vi "insertionSort.vi"() -> ()   [LabVIEW 2014]
panel:
  out "Insertion Sort":dbl[](graph)
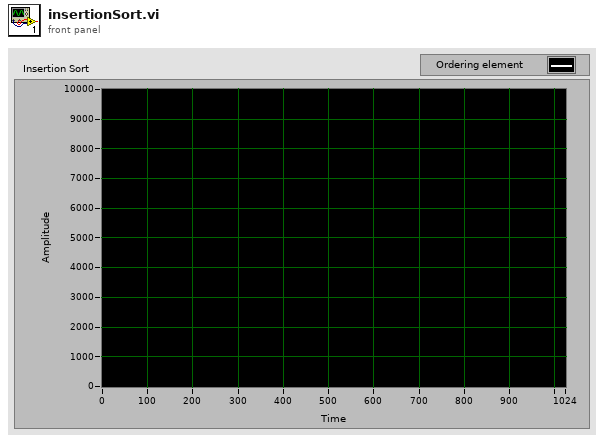
[diagram p1: front panel]
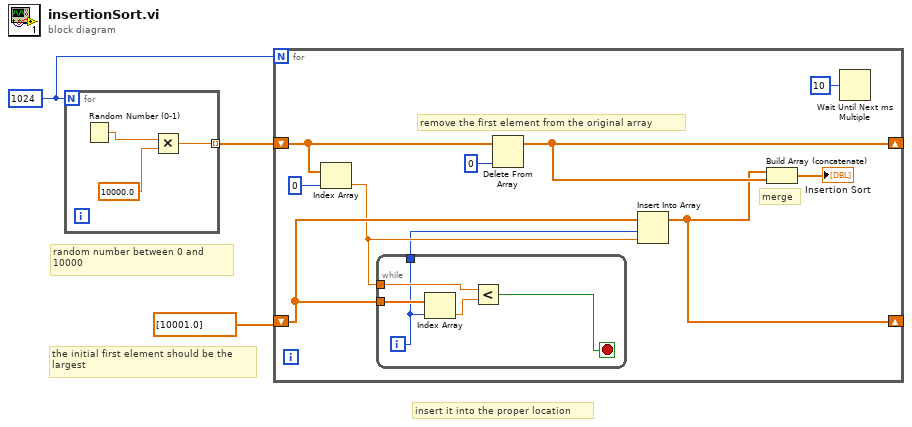
[diagram p0: block diagram]
diagram:
  w1 = 1024
  # "the initial first element should be the\nlargest"
  # "insert it into the proper location"
  # "random number between 0 and\n10000"
  n1 = for {
    N: w1 -> [_]
    tunnel: [w4] -> w3 mode=indexing
    n2 = Random Number (0-1)() -> (number: 0 to 1=w6:dbl)
    n3 = Multiply(x=w6, y=10000.0) -> (x*y=w4:dbl)
  }
  n4 = for {
    N: w1 -> [_]
    shift-right: [w10] -> _
    shift-left: w3 -> [w14]
    shift-right: [w7] -> _
    shift-left: dbl[] [10001.0] -> [w12]
    # "merge"
    # "remove the first element from the original array"
    n5 = Index Array(array=w14, index=0) -> (element=w11:dbl)
    n6 = while {
      tunnel: w12 -> [w21]
      tunnel: w11 -> [w19]
      tunnel: [w17] -> w8
      i -> [w17]
      stop <- w18 stop-if-true
      n7 = Index Array(array=w21, index=w17) -> (element=w20:dbl)
      n8 = Less?(x=w19, y=w20) -> (x < y?=w18:bool)
    }
    n9 = Delete From Array(array=w14, index=0) -> (array with subset deleted=w10:dbl[])  [unwired: 1 in, 1 out]
    n10 = Insert Into Array(array=w12, index=w8, new element=w11) -> (w7:dbl[])
    n11 = Build Array (concatenate)(w7, w10) -> (→"Insertion Sort":dbl[])
    n12 = Wait Until Next ms Multiple(millisecond multiple=u32 10 ("milliseconds to wait")) -> ()  [unwired: 1 out]
  }
